vi "DiffDriveTrainSim_New.vi"(6 "MeasurementStdDev":T2=[[0.0], [0.0], [0.0], [0.0], [0.0], [0.0], [0.0]], 7 "DriveTrainPlant":T1, 8 "WheelRadius_M":dbl, 9 "TrackWidth_M":dbl, 10 "Gearing":dbl=1.0, 11 "DriveMotor":T3 {"Jr_KgM2" format="%13.5p"; "L_H" format="%13.5p"; "Kt_NMPerAmp" format="%13.5p"; "KvINV_RadPerSecPerVolt" format="%13.5p"; "R_Ohms" format="%13.5p"; "FreeSpeed_RadPerSec" format="%13.5p"; "FreeCurrent_Amps" format="%13.5p"; "StallCurrent_Amps" format="%13.5p"; "StallTorque_NM" format="%13.5p"; "nominalVoltage_Volts" format="%13.5p"}) -> (3 "DiffDriveTrainSim":T4 {"m_Motor"."Jr_KgM2" format="%13.5p"; "m_Motor"."L_H" format="%13.5p"; "m_Motor"."Kt_NMPerAmp" format="%13.5p"; "m_Motor"."KvINV_RadPerSecPerVolt" format="%13.5p"; "m_Motor"."R_Ohms" format="%13.5p"; "m_Motor"."FreeSpeed_RadPerSec" format="%13.5p"; "m_Motor"."FreeCurrent_Amps" format="%13.5p"; "m_Motor"."StallCurrent_Amps" format="%13.5p"; "m_Motor"."StallTorque_NM" format="%13.5p"; "m_Motor"."nominalVoltage_Volts" format="%13.5p"})   [LabVIEW 2019, in "Trajectory_Library.lvlib"]
doc: "Create a SimDrivetrain .\n\nThis class simulates the state of the drivetrain. In simulationPeriodic, users should first set inputs from motors with setInputs(double, double)}, call update(double)} to update the simulation, and set estimated encoder and gyro positions, as well as estimated odometry pose. \n\nThe input linear state space system is:\nThe linear system is define as:\n - states\n - left velocity (m/s)\n - right velocity (m/s)\n - inputs\n - left voltage (volts)\n - right voltage(volts)\n - outputs\n - left velocity (m/s)\n - right velocity (m/s)\n\n \nOur state-space system is:\n \n x = [[x, y, theta, vel_l, vel_r, dist_l, dist_r]] \n\n in the field coordinate system (dist_* are wheel distances.)\n \n u = [[voltage_l, voltage_r]]? \n\n This is typically the control input of the last timestep from a LTVDiffDriveController.\n \n y = x\n \n\n \nInputs:\n - drivetrainPlant -- The LinearSystem representing the robot's drivetrain. This system can be created with LinearSystemId_createDrivetrainVelocitySystem(DCMotor, double, double, double, double, double)} or LinearSystemId_identifyDrivetrainSystem(double, double, double, double)}\n - driveMotor -- A DCMotor representing the drivetrain.\n - gearing -- The gearingRatio ratio of the robot, as output over input. This must be the same ratio as the ratio used to identify or create the drivetrainPlant.\n - trackWidthMeters -- The distance between the two sides of the drivetrian. Can be found with SysId.\n - wheelRadiusMeters -- The radius of the wheels on the drivetrain, in meters.\n - measurementStdDevs -- Standard deviations for measurements, in the form [x, y, heading, left velocity, right velocity, left distance, right distance]?. Can be null if no noise is desired. Gyro standard deviations of 0.0001 radians, velocity standard deviations of 0.05 m/s, and position measurement standard deviations of 0.005 meters are a reasonable starting point.\n\nOutputs:\n - OutDiffDriveTraimSim -- Updated data cluster."
uses:
  Trajectory_Library.lvlib
  TypeDef/DIFF_DRIVE_TRAIN_SIM.ctl
  TypeDef/LINEAR_SYSTEM.ctl
  <vilib>/Analysis/Matrix/Datatypes/RealMatrix.ctl
  TypeDef/DCMOTOR.CTL
  <vilib>/Analysis/Matrix/NI_Matrix.lvlib
panel:
  # "<1, 1>"
  # "<States,States>"
  # "<States,Inputs>"
  # "<Outputs,States>"
  # "<Outputs,Inputs>"
  # "<States, 1>"
  # "<Outputs, 1>"
  # "<Inputs, 1>"
  # "<Outputs, 1>"
  # "<States,States>"
  # "<States,Inputs>"
  # "<Outputs,States>"
  # "<Outputs,Inputs>"
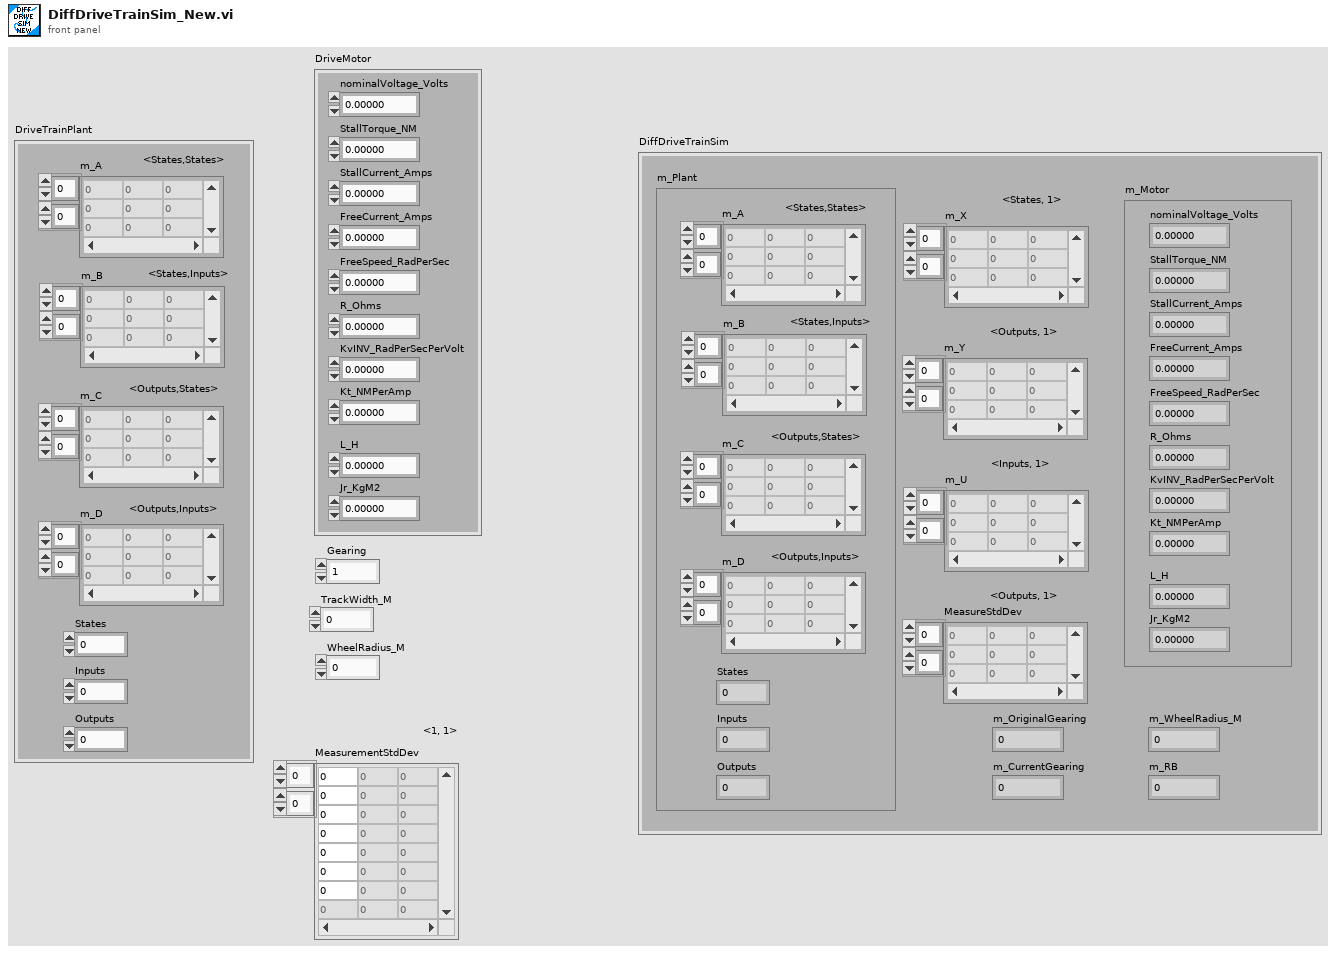
[diagram p1: front panel]
types:
  T1 = typedef "Trajectory_Library.lvlib/LINEAR_SYSTEM.ctl" = cluster{"m_A":T2, "m_B":T2, "m_C":T2, "m_D":T2, "States":i32, "Inputs":i32, "Outputs":i32}
  T2 = typedef "NI_Matrix.lvlib/RealMatrix.ctl" = dbl[][]
  T3 = typedef "Trajectory_Library.lvlib/DCMOTOR.CTL" = cluster{"nominalVoltage_Volts":dbl, "StallTorque_NM":dbl, "StallCurrent_Amps":dbl, "FreeCurrent_Amps":dbl, "FreeSpeed_RadPerSec":dbl, "R_Ohms":dbl, "KvINV_RadPerSecPerVolt":dbl, "Kt_NMPerAmp":dbl, "L_H":dbl, "Jr_KgM2":dbl}
  T4 = typedef "Trajectory_Library.lvlib/DIFF_DRIVE_TRAIN_SIM.ctl" = cluster{"m_Plant":T1, "m_X":T2, "m_Y":T2, "m_U":T2, "MeasureStdDev":T2, "m_Motor":T3, "m_OriginalGearing":dbl, "m_CurrentGearing":dbl, "m_WheelRadius_M":dbl, "m_RB":dbl}
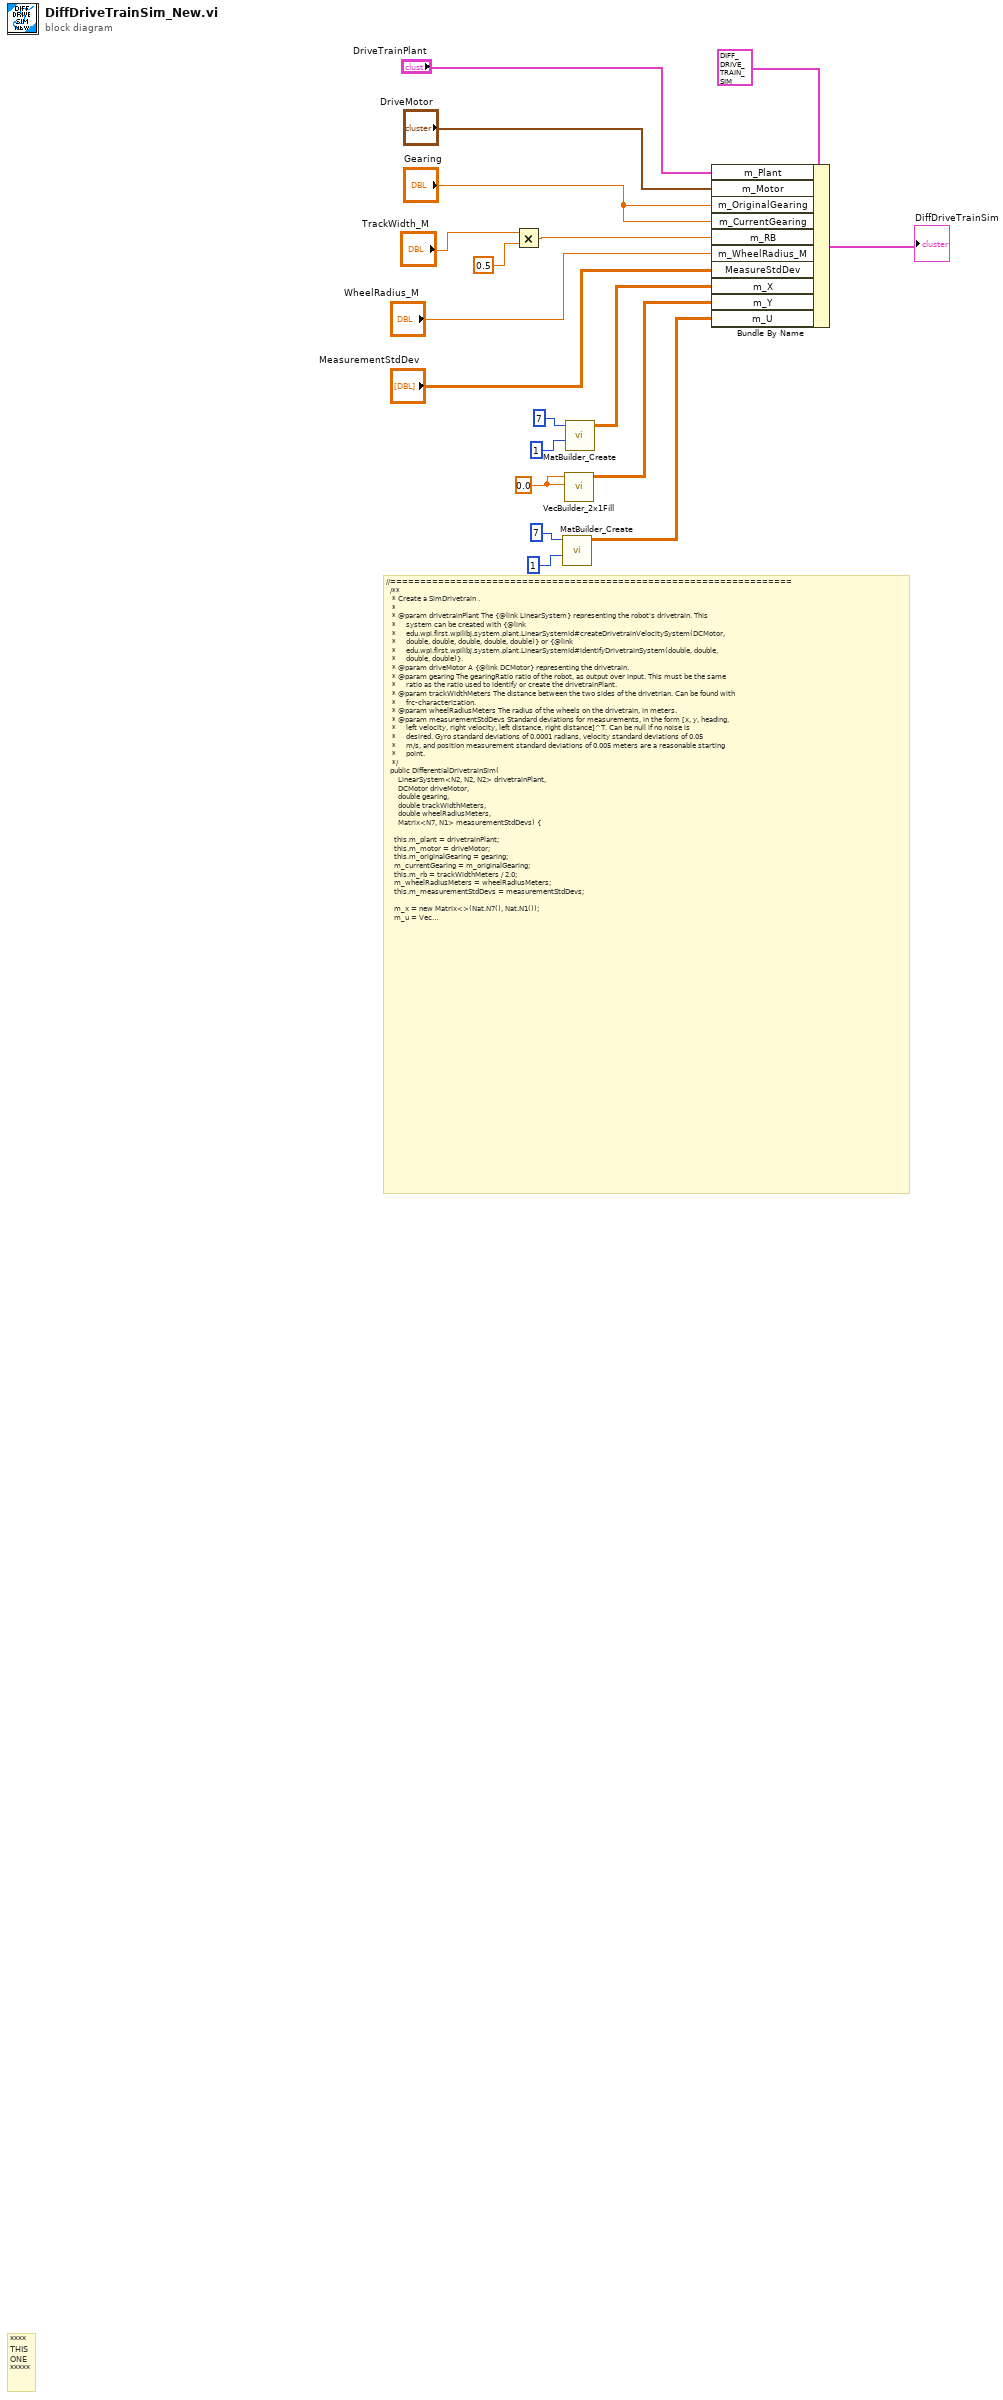
[diagram p0: block diagram]
diagram:
  w4 = 0.0 ("R0")
  # "//===================================================================\n  /**\n   * Create a SimDrivetrain .\n   *\n   * @param drivetrainPlant The {@link LinearSystem} representing the robot's drivetrain. This\n   *     system can be created with {@link\n   *     edu.wpi.first.wpilibj.system.plant.LinearSystemId#createDrivetrainVelocitySystem(DCMotor,\n   *     double, double, double, double, double)} or {@link\n   *     edu.wpi.first.wpilibj.system.plant.LinearSystemId#identifyDrivetrainSystem(double, double,\n   *     double, double)}.\n   * @param driveMotor A {@link DCMotor} representing the drivetrain.\n   * @param gearing The gearingRatio ratio of the robot, as output over input. This must be the same\n   *     ratio as the ratio used to identify or create the drivetrainPlant.\n   * @param trackWidthMeters The distance between the two sides of the drivetrian. Can be found with\n   *     frc-characterization.\n   * @param wheelRadiusMeters The radius of the wheels on the drivetrain, in meters.\n   * @param measurementStdDevs Standard deviations for measurements, in the form [x, y, heading,\n   *     left velocity, right velocity, left distance, right distance]^T. Can be null if no noise is\n   *     desired. Gyro standard deviations of 0.0001 radians, velocity standard deviations of 0.05\n   *     m/s, and position measurement standard deviations of 0.005 meters are a reasonable starting\n   *     point.\n   */\n  public DifferentialDrivetrainSim(\n      LinearSystem<N2, N2, N2> drivetrainPlant,\n      DCMotor driveMotor,\n      double gearing,\n      double trackWidthMeters,\n      double wheelRadiusMeters,\n      Matrix<N7, N1> measurementStdDevs) {\n\n    this.m_plant = drivetrainPlant;\n    this.m_motor = driveMotor;\n    this.m_originalGearing = gearing;\n    m_currentGearing = m_originalGearing;\n    this.m_rb = trackWidthMeters / 2.0;\n    m_wheelRadiusMeters = wheelRadiusMeters;\n    this.m_measurementStdDevs = measurementStdDevs;\n\n    m_x = new Matrix<>(Nat.N7(), Nat.N1());\n    m_u = VecBuilder.fill(0, 0);\n    m_y = new Matrix<>(Nat.N7(), Nat.N1());\n  }"
  # "****\nTHIS\nONE\n*****"
  n1 = Multiply(x="TrackWidth_M", y=0.5) -> (x*y=w10:dbl)
  n2 = call "MatBuilder_Create.vi"("Columns"=1, "Rows"=7) -> ("output matrix"=w1:T2)  [unwired: 9 in]
  n3 = call "VecBuilder_2x1Fill.vi"("R1"=w4, "R0"=w4) -> ("output matrix"=w2:T2)  [unwired: 9 in]
  n4 = call "MatBuilder_Create.vi"("Columns"=1, "Rows"=7) -> ("output matrix"=w3:T2)  [unwired: 9 in]
  n5 = Bundle By Name(cluster=T4 {"m_Plant"={"m_A"=[], "m_B"=[], "m_C"=[], "m_D"=[], "States"=0, "Inputs"=0, "Outputs"=0}, "m_X"=[], "m_Y"=[], "m_U"=[], "MeasureStdDev"=[], "m_Motor"={"nominalVoltage_Volts"=0.0, "StallTorque_NM"=0.0, "StallCurrent_Amps"=0.0, "FreeCurrent_Amps"=0.0, "FreeSpeed_RadPerSec"=0.0, "R_Ohms"=0.0, "KvINV_RadPerSecPerVolt"=0.0, "Kt_NMPerAmp"=0.0, "L_H"=0.0, "Jr_KgM2"=0.0}, "m_OriginalGearing"=0.0, "m_CurrentGearing"=0.0, "m_WheelRadius_M"=0.0, "m_RB"=0.0} ("DIFF_DRIVE_TRAIN_SIM"), "m_Plant"="DriveTrainPlant", "m_Motor"="DriveMotor", "m_OriginalGearing"="Gearing", "m_CurrentGearing"="Gearing", "m_RB"=w10, "m_WheelRadius_M"="WheelRadius_M", "MeasureStdDev"="MeasurementStdDev", "m_X"=w3, "m_Y"=w2, "m_U"=w1) -> (→"DiffDriveTrainSim":T4)
